vi "test17.1-RegisterStatesFromNonCSM_State.vi"(8 "error in (no error)":errorcluster, 11 "TestCase in":refnum<class "testcase-CSMBroadcast.lvclass">) -> (0 "error out":errorcluster, 3 "TestCase out":refnum<class "testcase-CSMBroadcast.lvclass">)   [LabVIEW 2017, in "testcase-CSMBroadcast.lvclass"]
uses:
  testcase-CSMBroadcast.lvclass
  <vilib>/addons/_JKI Toolkits/VI Tester/TestCase.llb/TestCase.lvclass
  src/user.lib/_NEVSTOP/Communicable State Machine(CSM)/Communicable State Machine.lvlib
  C:/Program Files (x86)/National Instruments/LabVIEW 2017/vi.lib/addons/_JKI Toolkits/VI Tester/TestCase.llb/TestCase.lvclass
panel:
  out "error out 3":errorcluster
  out "error out 2":errorcluster
  out "LoopCount":i32
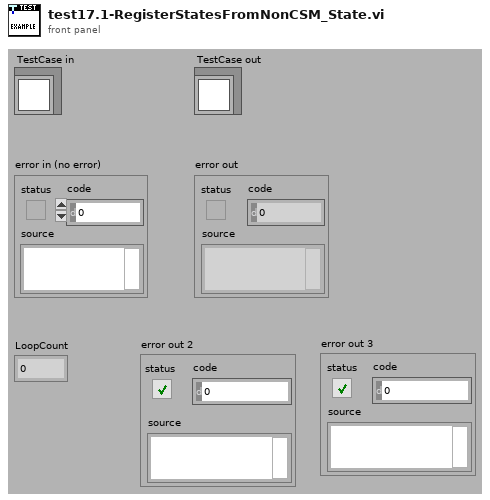
[diagram p1: front panel]
types:
  T1 = cluster{"ModuleName":string, "Status":string, "Arguments":string}
  T2 = cluster{"cluster":cluster{"ModuleName":string, "Status":string, "Arguments":string}}
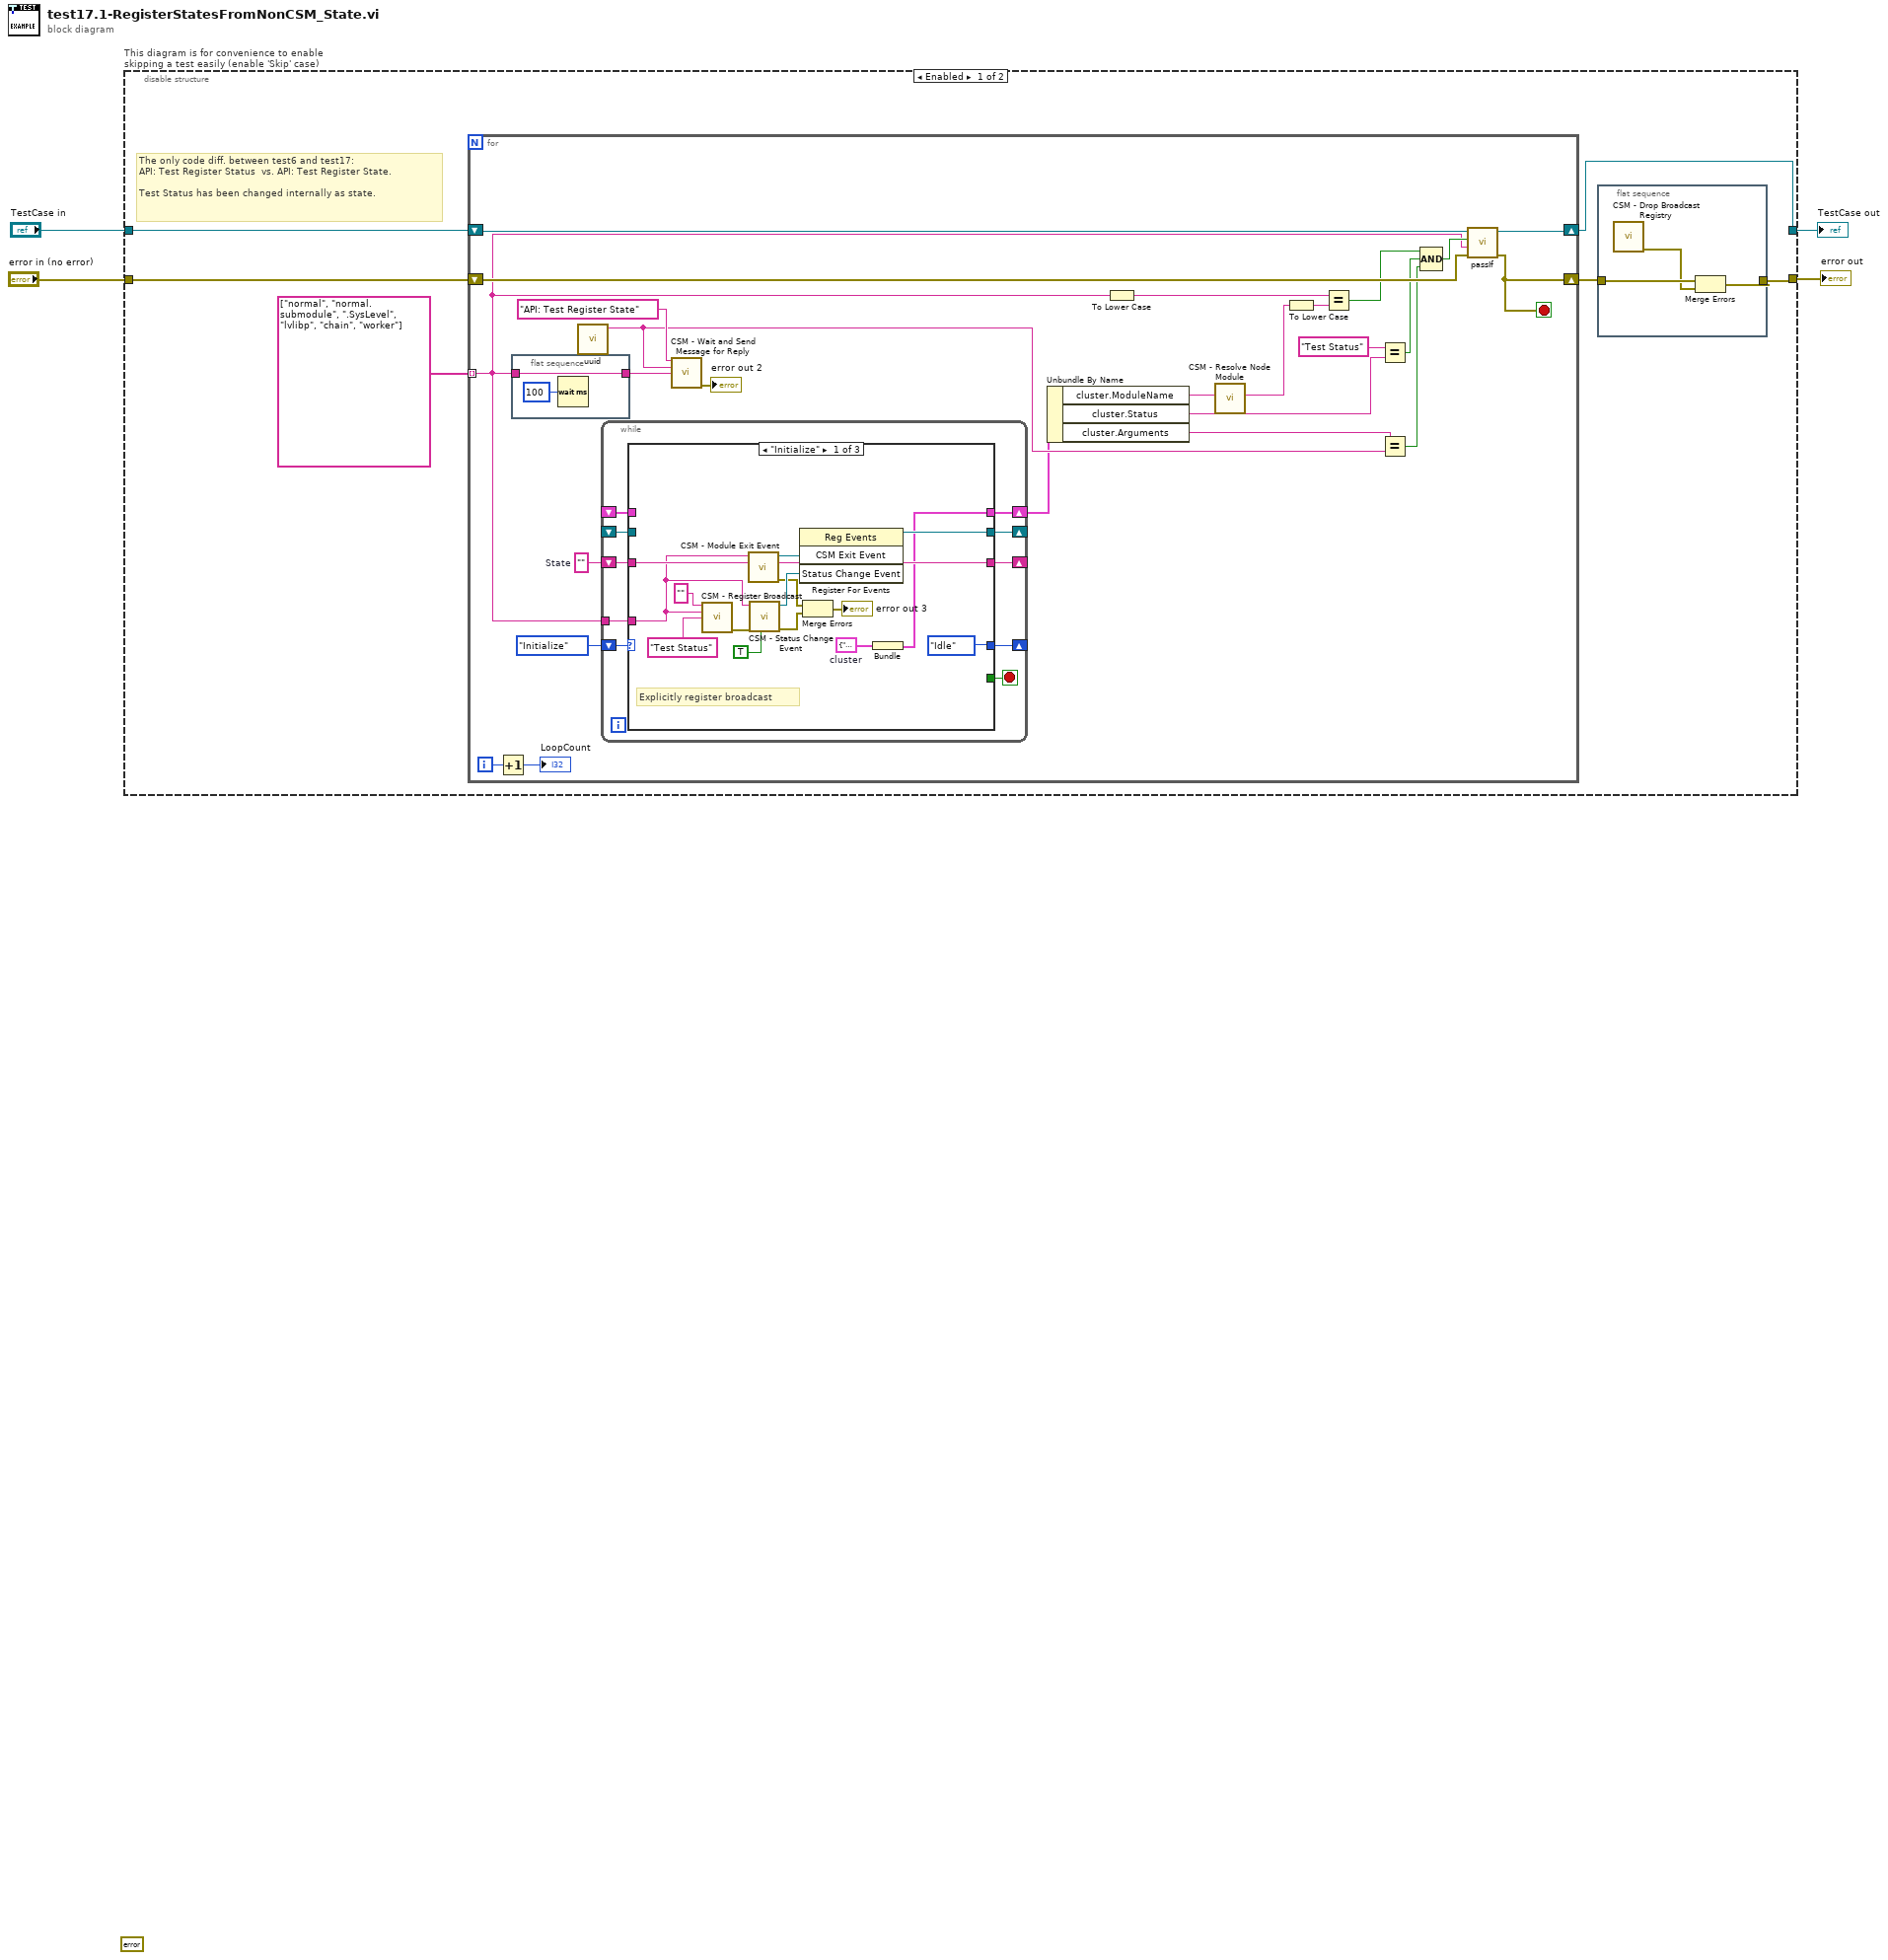
[diagram p0: block diagram]
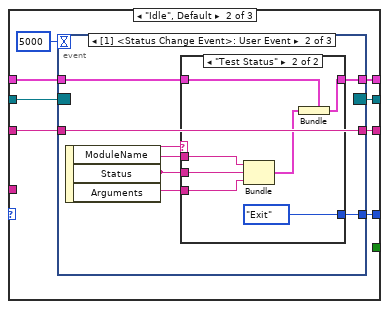
[diagram p2: hidden frame]
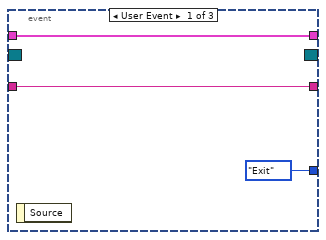
[diagram p3: hidden frame]
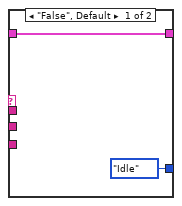
[diagram p4: hidden frame]
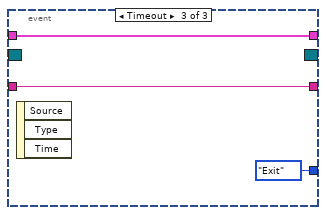
[diagram p5: hidden frame]
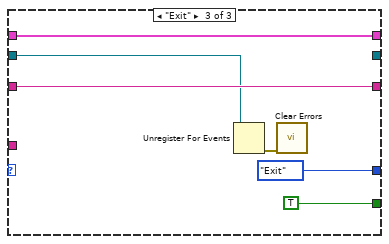
[diagram p6: hidden frame]
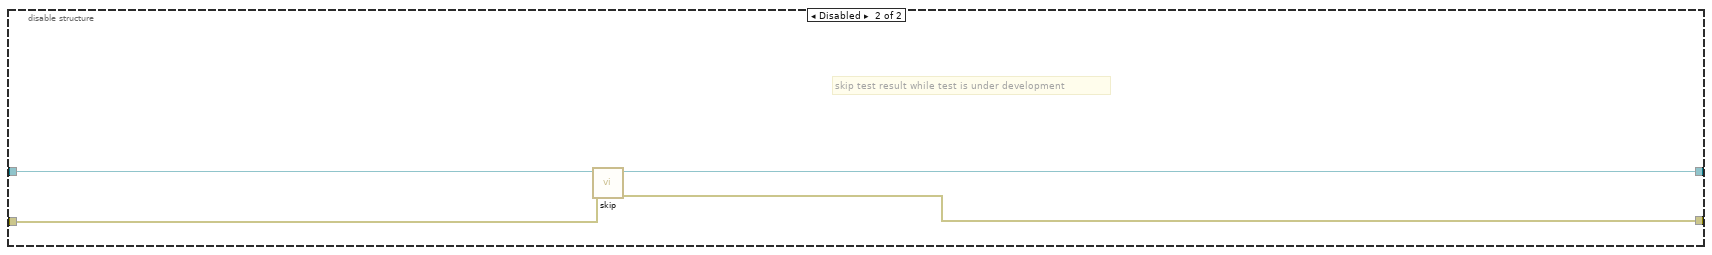
[diagram p7: hidden frame]
diagram:
  (unwired) errorcluster {"status"=FALSE, "code"=0, "source"=""} ("error out")
  n1 = disable-structure "This diagram is for convenience to enable skipping a test easily (enable 'Skip' case)" shown="Enabled" {
    disable-tunnel: "TestCase in" -> [w10 w105]
    disable-tunnel: [w6 w103] -> w2
    disable-tunnel: [w5 w104] -> w1
    disable-tunnel: "error in (no error)" -> [w9 w102]
    frame Enabled {
      # "The only code diff. between test6 and test17:\nAPI: Test Register Status  vs. API: Test Register State.\n\nTest Status has been changed internally as state."
      n2 = for {
        shift-right: [w29] -> w6
        shift-left: w10 -> [w30]
        shift-right: [w20] -> w7
        shift-left: w9 -> [w28]
        tunnel: string[] ["normal", "normal.submodule", ".SysLevel", "lvlibp", "chain", "worker"] -> [w15] mode=indexing
        i -> [w23]
        stop <- w20 stop-if-true
        w37 = ""  # State
        n3 = Increment(x=w23) -> (x+1=→"LoopCount":i32)
        n4 = flat-sequence {
          tunnel: w15 -> [w40]
          tunnel: [w40] -> w35
          frame #0 {
            n5 = Wait (ms)(milliseconds to wait=u32 100) -> ()  [unwired: 1 out]
          }
        }
        n6 = call "uuid.vi"() -> ("UUID"=w32:string)  [unwired: 11 in]
        n7 = while {
          shift-right: [w49] -> _
          shift-left: enum16{"Idle", "Initialize", "Exit"}."Initialize" -> [w50]
          shift-right: [w46] -> _
          shift-left: w37 -> [w47]
          shift-right: [w45] -> _
          shift-left: _ -> [w44]
          shift-right: [w43] -> w19
          shift-left: _ -> [w42]
          tunnel: w15 -> [w41]
          stop <- w48 stop-if-true
          n8 = case shown="\"Initialize\"" w50 {
            tunnel: [enum16{"Idle", "Initialize", "Exit"}."Idle" w73 enum16{"Idle", "Initialize", "Exit"}."Exit"] -> w49
            tunnel: [_ _ TRUE] -> w48
            tunnel: w47 -> [w64 w71 w99]
            tunnel: [w64 w72 w99] -> w46
            tunnel: [w62 w69 _] -> w45
            tunnel: w44 -> [_ w70 w98]
            tunnel: [w61 w67 w96] -> w43
            tunnel: w42 -> [_ w68 w96]
            tunnel: w41 -> [w54 _ _]
            frame "Initialize" {
              w59 = T1 {"ModuleName"="", "Status"="", "Arguments"=""}  # cluster
              # "Explicitly register broadcast"
              n9 = call "CSM - Register Broadcast.vi"("CSM Name(Empty for Broadcast Event)"="", "Source CSM Name (* as Default)"=w54, "Trigger"="Test Status" ("State")) -> ("error out"=w55:errorcluster)  [unwired: 11 in, 1 out]
              n10 = call "CSM - Module Exit Event.vi"("Name (\"\" to Use UUID) In"=w54) -> ("error out"=w58:errorcluster, "CSM Exit Event"=w63:refnum<user-event>)  [unwired: 8 in, 1 out]
              n11 = call "CSM - Status Change Event.vi"("Auto Register? (T)"=TRUE, "Error In"=w55, "CSM Module"=w54) -> ("error out"=w57:errorcluster, "Status Change Event"=w60:refnum<user-event>)  [unwired: 6 in, 1 out]
              n12 = register-events(w63, w60) -> (reference out=w62:refnum<event-registration>)  [unwired: 2 in, 1 out]
              n13 = Merge Errors(w58, w57) -> (→"error out 3":errorcluster)
              n14 = Bundle("cluster"=w59) -> (w61:T2)  [unwired: 1 in]
            }
            frame "Idle", Default {
              n15 = event shown="[1] <Status Change Event>: User Event" {
                selector: w70 -> [_ _ _]
                dyn-events: [_ _ _] -> w69
                timeout: 5000 -> [_ _ _]
                tunnel: [enum16{"Idle", "Initialize", "Exit"}."Exit" w82 enum16{"Idle", "Initialize", "Exit"}."Exit"] -> w73
                tunnel: w71 -> [w76 w83 w95]
                tunnel: [w76 w83 w95] -> w72
                tunnel: w68 -> [w74 w79 w94]
                tunnel: [w74 w78 w94] -> w67
                event User Event {
                  n16 = event-data() -> ()  [unwired: 1 in, 1 out]
                }
                event User Event {
                  n17 = event-data() -> ("ModuleName"=w81:string, "Status"=w77:string, "Arguments"=w80:string)  [unwired: 1 in]
                  n18 = case shown="\"Test Status\"" w77 {
                    tunnel: [enum16{"Idle", "Initialize", "Exit"}."Idle" enum16{"Idle", "Initialize", "Exit"}."Exit"] -> w82
                    tunnel: w81 -> [_ w91]
                    tunnel: w77 -> [_ w90]
                    tunnel: w80 -> [_ w89]
                    tunnel: w79 -> [w85 w88]
                    tunnel: [w85 w86] -> w78
                    frame "False", Default {
                    }
                    frame "Test Status" {
                      n19 = Bundle("ModuleName"=w91, "Status"=w90, "Arguments"=w89) -> (w87:T1)  [unwired: 1 in]
                      n20 = Bundle(cluster=w88, "cluster"=w87) -> (w86:T2)
                    }
                  }
                }
                event Timeout {
                  n21 = event-data() -> ()  [unwired: 1 in, 3 out]
                }
              }
            }
            frame "Exit" {
              n22 = Unregister For Events(event registration refnum=w98) -> (error out=w97:errorcluster)  [unwired: 1 in]
              n23 = call <vilib>:"Clear Errors.vi"("error in (no error)"=w97) -> ()  [unwired: 5 in, 2 out]
            }
          }
        }
        n24 = call "CSM - Wait and Send Message for Reply.vi"("State"="API: Test Register State", "Arguments (\"\")"=w32, "Target Module"=w35) -> ("error out"=→"error out 2":errorcluster)  [unwired: 9 in, 3 out]
        n25 = Unbundle By Name(w19) -> ("cluster.ModuleName"=w17:string, "cluster.Status"=w33:string, "cluster.Arguments"=w31:string)
        n26 = To Lower Case(string=w15) -> (all lower case string=w18:string)
        n27 = call "CSM - Resolve Node Module.vi"("Node Name"=w17) -> ("CSM Module Name"=w14:string)  [unwired: 10 in]
        n28 = To Lower Case(string=w14) -> (all lower case string=w16:string)
        n29 = Equal?(x=w18, y=w16) -> (x = y?=w27:bool)
        n30 = Equal?(x="Test Status" ("State"), y=w33) -> (x = y?=w26:bool)
        n31 = Equal?(x=w31, y=w32) -> (x = y?=w25:bool)
        n32 = Compound Arithmetic op=AND(w27, w26, w25) -> (w24:bool)
        n33 = call-dynamic "passIf.vi"("error in (no error)"=w28, "message (\"\")"=w15, "pass"=w24, "TestCase in"=w30) -> ("error out"=w20:errorcluster, "TestCase out"=w29:refnum<class "testcase-CSMBroadcast.lvclass">)  [unwired: 6 in]
      }
      n34 = flat-sequence {
        tunnel: w7 -> [w13]
        tunnel: [w12] -> w5
        frame #0 {
          n35 = call "CSM - Drop Broadcast Registry.vi"() -> ("error out"=w11:errorcluster)  [unwired: 15 in]
          n36 = Merge Errors(w13, w11) -> (w12:errorcluster)
        }
      }
    }
    frame Disabled {
      # "skip test result while test is under development"
      n37 = call <vilib>:"skip.vi"("error in (no error)"=w102, "TestCase in"=w105) -> ("error out"=w104:errorcluster, "TestCase out"=w103:refnum<class "testcase-CSMBroadcast.lvclass">)  [unwired: 8 in]
    }
  }
  "error out" <- w1
  "TestCase out" <- w2
